vi "Main.vi"() -> ()   [LabVIEW 2015]
doc: "This template is for the Queued Message Handler design pattern.\n\nThe Event Handling Loop generates messages based on user interface actions.\n\nThe Message Handling Loop processes messages generated by the Event Handling Loop, or by other messages. The messages are string values, so new messages can be added easily to the Message Cases case structure in the Message Handling Loop. Each message cluster can also provide an optional value for Message Data, which is a variant that can be converted to whatever message-specific data is required."
uses:
  controls/UI Data.ctl
  support/Message Queue/Message Queue.lvlib
  support/User Event - Stop/User Event - Stop.lvlib
panel:
  out "Display <Replace Me>":string
  in  "Do Something Else <Replace Me>":bool
  in  "Do Something <Replace Me>":bool
  in  "Stop Button":bool
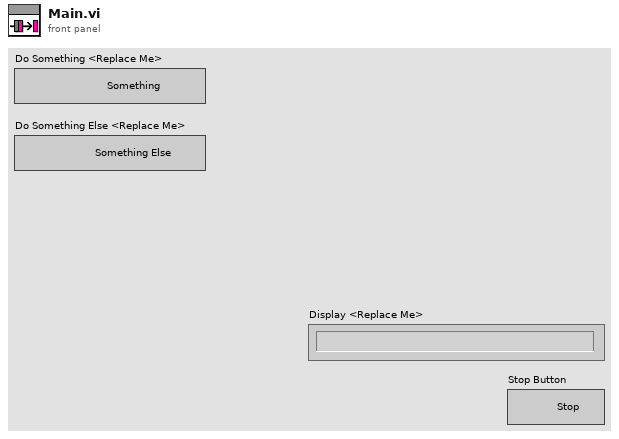
[diagram p1: front panel]
types:
  T1 = typedef "UI Data.ctl" = cluster{"Boolean <Replace Me>":bool, "String <Replace Me>":string, "Numeric <Replace Me>":dbl, "Do Something Ref":refnum<vi>, "Do Something Else Ref":refnum<vi>, "Data Display Ref":refnum<vi>, "Stop Button Ref":refnum<vi>}
  T2 = typedef "Message Queue.lvlib/All Message Queues.ctl" = cluster{"MHL":refnum<queue>, "Boiler controller":refnum<queue>}
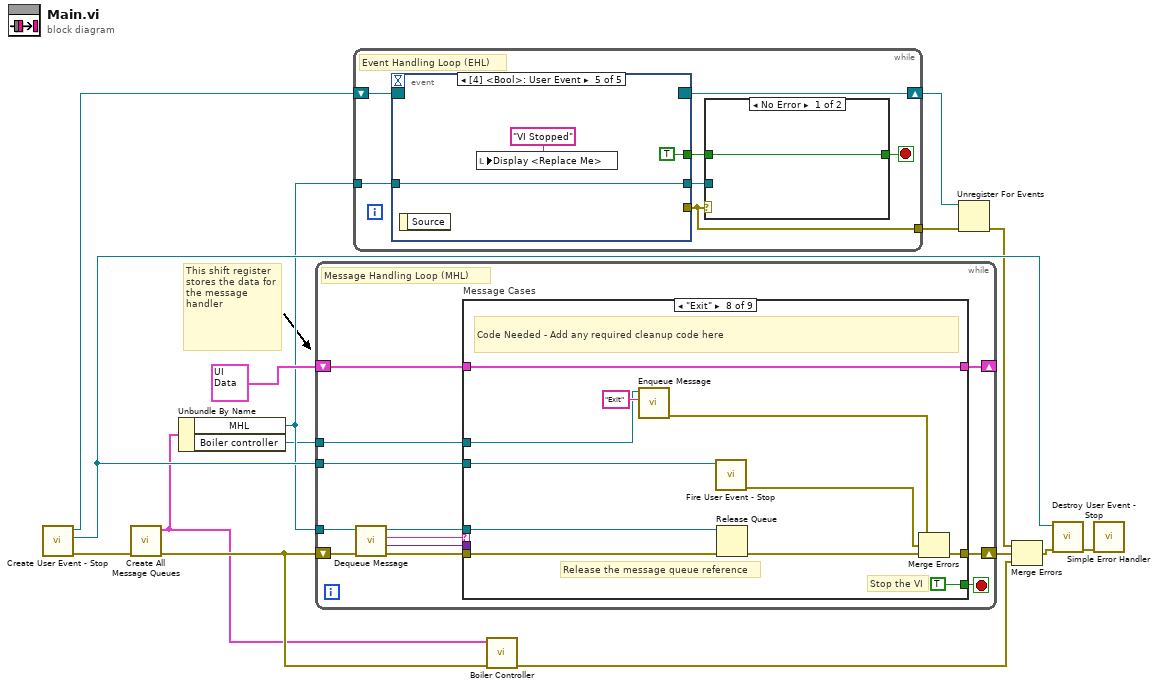
[diagram p0: block diagram]
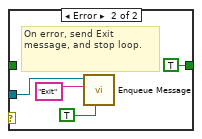
[diagram p2: hidden frame]
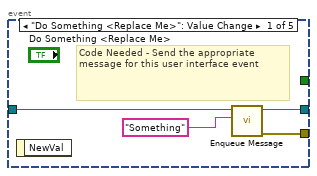
[diagram p3: hidden frame]
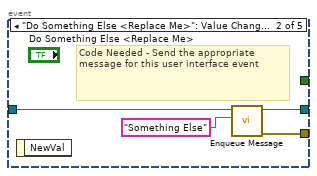
[diagram p4: hidden frame]
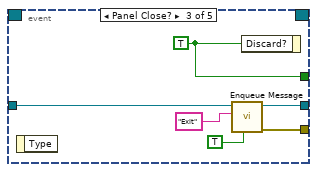
[diagram p5: hidden frame]
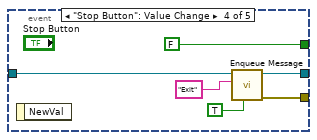
[diagram p6: hidden frame]
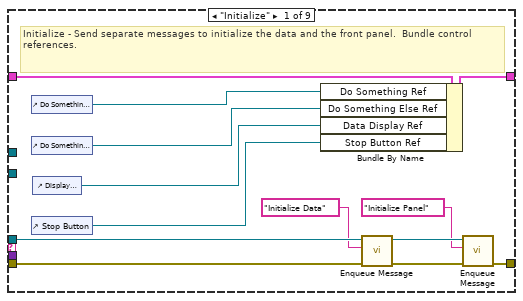
[diagram p7: hidden frame]
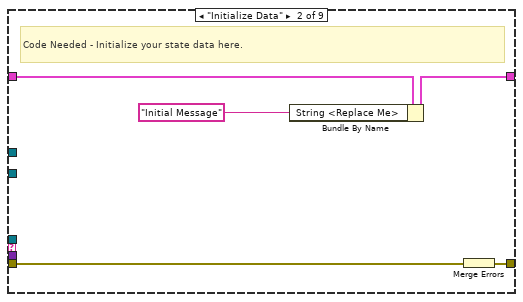
[diagram p8: hidden frame]
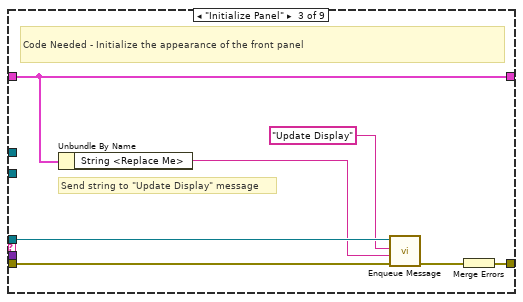
[diagram p9: hidden frame]
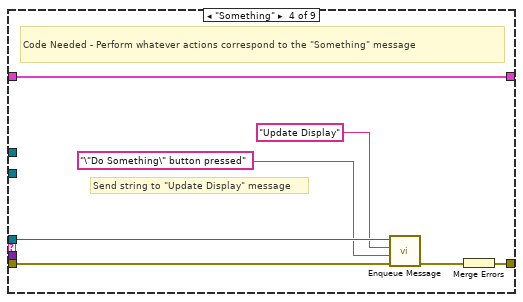
[diagram p10: hidden frame]
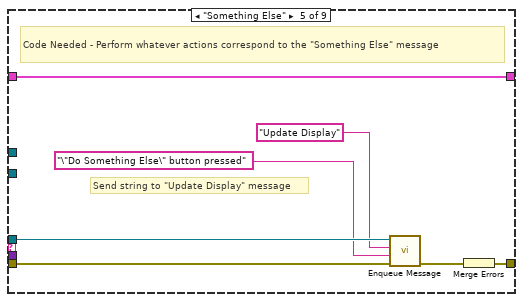
[diagram p11: hidden frame]
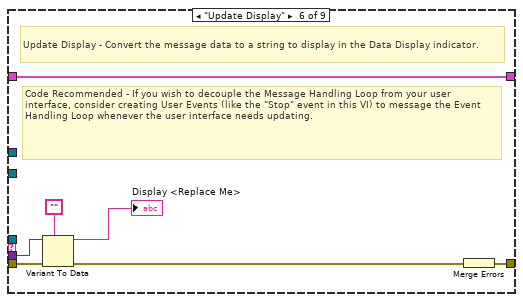
[diagram p12: hidden frame]
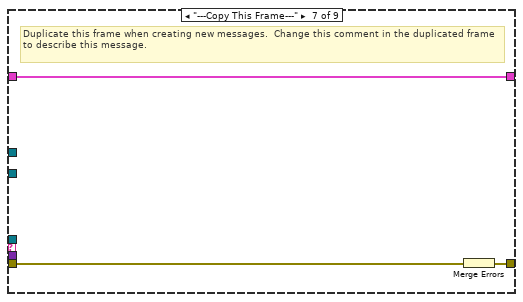
[diagram p13: hidden frame]
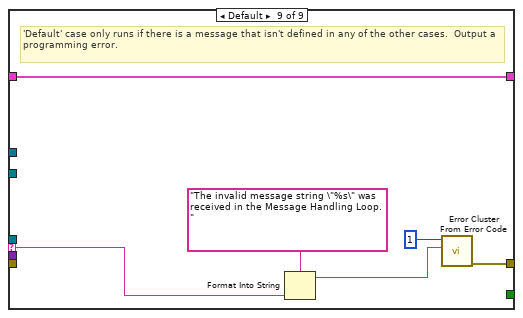
[diagram p14: hidden frame]
diagram:
  # "This shift register\nstores the data for the message handler"
  n1 = call "Create User Event - Stop.vi"() -> ("error out"=w14:errorcluster, "User bool - Stop"=w11:refnum<user-event>, "Event Registration Refnum"=w6:refnum<event-registration>)  [unwired: 9 in]
  n2 = call "Create All Message Queues.vi"("error in (no error)"=w14) -> ("error out"=w5:errorcluster, "Message Queues out"=w2:T2)  [unwired: 9 in]
  n3 = Unbundle By Name(w2) -> ("MHL"=w4:refnum<queue>, "Boiler controller"=w3:refnum<queue>)
  n4 = while {
    tunnel: w4 -> [w17]
    shift-right: [w26] -> _
    shift-left: T1 {"Boolean <Replace Me>"=TRUE, "String <Replace Me>"="", "Numeric <Replace Me>"=0.0, "Do Something Ref"=refnum, "Do Something Else Ref"=refnum, "Data Display Ref"=refnum, "Stop Button Ref"=refnum} ("Data Cluster") -> [w27]
    tunnel: w11 -> [w23]
    shift-right: [w24] -> w15
    shift-left: w5 -> [w22]
    tunnel: w3 -> [w16]
    stop <- w25 stop-if-true
    # "Message Handling Loop (MHL)"
    n5 = call "Dequeue Message.vi"("error in (no error)"=w22, "Message Queue"=w17) -> ("error out"=w21:errorcluster, "Message Data"=w19:variant, "Message"=w20:string, "dup Message Queue"=w18:refnum<queue>)  [unwired: 6 in]
    n6 = case "Message Cases" shown="\"Exit\"" w20 {
      selector: w20 -> [_ _ _ _ _ _ _ _ w91]
      tunnel: w18 -> [w36 _ w49 w55 w62 _ _ w87 _]
      tunnel: w21 -> [w39 w45 w50 w57 w64 w71 w76 w82 _]
      tunnel: [w40 w41 w51 w58 w65 w72 w74 w83 w89] -> w24
      tunnel: w27 -> [w33 w44 w52 w59 w66 w73 w75 w86 w93]
      tunnel: [w32 w43 w52 w59 w66 w73 w75 w86 w93] -> w26
      tunnel: [_ _ _ _ _ _ _ TRUE _] -> w25
      tunnel: w19 -> [_ _ _ _ _ w70 _ _ _]
      tunnel: w23 -> [_ _ _ _ _ _ _ w81 _]
      tunnel: w16 -> [_ _ _ _ _ _ _ w78 _]
      frame "Initialize" {
        # "Initialize - Send separate messages to initialize the data and the front panel.  Bundle control references."
        n7 = control-ref of="Do Something <Replace Me>"() -> (w31:refnum<vi>)
        n8 = control-ref of="Do Something Else <Replace Me>"() -> (w30:refnum<vi>)
        n9 = control-ref of="Stop Button"() -> (w28:refnum<vi>)
        n10 = control-ref of="Display <Replace Me>"() -> (w29:refnum<vi>)
        n11 = Bundle By Name(cluster=w33, "Do Something Ref"=w31, "Do Something Else Ref"=w30, "Data Display Ref"=w29, "Stop Button Ref"=w28) -> (w32:T1)
        n12 = call "Enqueue Message.vi"("error in (no error)"=w39, "Message"="Initialize Data", "Message Queue"=w36) -> ("error out"=w38:errorcluster, "dup Message Queue"=w37:refnum<queue>)  [unwired: 7 in]
        n13 = call "Enqueue Message.vi"("error in (no error)"=w38, "Message"="Initialize Panel", "Message Queue"=w37) -> ("error out"=w40:errorcluster)  [unwired: 7 in, 1 out]
      }
      frame "Initialize Data" {
        # "Code Needed - Initialize your state data here."
        n14 = Bundle By Name(cluster=w44, "String <Replace Me>"="Initial Message" ("Initial Message")) -> (w43:T1)
        n15 = Merge Errors(w45) -> (w41:errorcluster)
      }
      frame "Initialize Panel" {
        # "Send string to \"Update Display\" message"
        # "Code Needed - Initialize the appearance of the front panel"
        n16 = Unbundle By Name(w52) -> ("String <Replace Me>"=w46:string)
        n17 = call "Enqueue Message.vi"("error in (no error)"=w50, "Message Data"=w46, "Message"="Update Display", "Message Queue"=w49) -> ("error out"=w48:errorcluster)  [unwired: 6 in, 1 out]
        n18 = Merge Errors(w48) -> (w51:errorcluster)
      }
      frame "Something" {
        # "Send string to \"Update Display\" message"
        # "Code Needed - Perform whatever actions correspond to the \"Something\" message"
        n19 = call "Enqueue Message.vi"("error in (no error)"=w57, "Message Data"="\"Do Something\" button pressed" ("\"Do Something\" button pressed"), "Message"="Update Display", "Message Queue"=w55) -> ("error out"=w56:errorcluster)  [unwired: 6 in, 1 out]
        n20 = Merge Errors(w56) -> (w58:errorcluster)
      }
      frame "Something Else" {
        # "Send string to \"Update Display\" message"
        # "Code Needed - Perform whatever actions correspond to the \"Something Else\" message"
        n21 = call "Enqueue Message.vi"("error in (no error)"=w64, "Message Data"="\"Do Something Else\" button pressed" ("\"Do Something Else\" button pressed"), "Message"="Update Display", "Message Queue"=w62) -> ("error out"=w63:errorcluster)  [unwired: 6 in, 1 out]
        n22 = Merge Errors(w63) -> (w65:errorcluster)
      }
      frame "Update Display" {
        # "Code Recommended - If you wish to decouple the Message Handling Loop from your user interface, consider creating User Events (like the \"Stop\" event in this VI) to message the Event Handling Loop whenever the user interface needs updating."
        # "Update Display - Convert the message data to a string to display in the Data Display indicator."
        n23 = Variant To Data(error in=w71, type="", Variant=w70) -> (data=→"Display <Replace Me>":string, error out=w68:errorcluster)
        n24 = Merge Errors(w68) -> (w72:errorcluster)
      }
      frame "---Copy This Frame---" {
        # "Duplicate this frame when creating new messages.  Change this comment in the duplicated frame to describe this message."
        n25 = Merge Errors(w76) -> (w74:errorcluster)
      }
      frame "Exit" {
        # "Stop the VI"
        # "Release the message queue reference"
        # "Code Needed - Add any required cleanup code here"
        n26 = call "Enqueue Message.vi"("Message"="Exit", "Message Queue"=w78) -> ("error out"=w77:errorcluster)  [unwired: 8 in, 1 out]
        n27 = call "Fire User Event - Stop.vi"("User Event - Stop"=w81) -> ("error out"=w80:errorcluster)  [unwired: 10 in]
        n28 = Release Queue(queue=w87, error in (no error)=w82) -> (error out=w84:errorcluster)  [unwired: 1 in, 2 out]
        n29 = Merge Errors(w77, w80, w84) -> (w83:errorcluster)
      }
      frame Default {
        # "'Default' case only runs if there is a message that isn't defined in any of the other cases.  Output a programming error."
        n30 = Format Into String(format string="The invalid message string \"%s\" was received in the Message Handling Loop." ("Unknown Message Error Text"), w91) -> (resulting string=w88:string)  [unwired: 2 in, 1 out]
        n31 = call <vilib>:"Error Cluster From Error Code.vi"("error message (\"\")"=w88, "error code (0)"=1) -> ("error out"=w89:errorcluster)  [unwired: 7 in]
      }
    }
  }
  n32 = while {
    tunnel: w4 -> [w100]
    tunnel: [w96] -> w9
    shift-right: [w95] -> w8
    shift-left: w6 -> [w94]
    stop <- w98 stop-if-true
    # "Event Handling Loop (EHL)"
    n33 = event shown="[4] <Bool>: User Event" {
      selector: w94 -> [_ _ _ _ _]
      dyn-events: [_ _ _ _ _] -> w95
      timeout: _ -> [_ _ _ _ _]
      tunnel: [_ _ w119 FALSE ("Discard?") TRUE ("Discard?")] -> w99
      tunnel: w100 -> [w109 w113 w118 w125 w128]
      tunnel: [w108 w111 w117 w124 _] -> w96
      tunnel: [w107 w112 w116 w122 w128] -> w97
      event "Do Something <Replace Me>": Value Change {
        # "Code Needed - Send the appropriate message for this user interface event"
        n34 = event-data() -> ()  [unwired: 1 in, 1 out]
        n35 = call "Enqueue Message.vi"("Message"="Something", "Message Queue"=w109) -> ("error out"=w108:errorcluster, "dup Message Queue"=w107:refnum<queue>)  [unwired: 8 in]
      }
      event "Do Something Else <Replace Me>": Value Change {
        # "Code Needed - Send the appropriate message for this user interface event"
        n36 = event-data() -> ()  [unwired: 1 in, 1 out]
        n37 = call "Enqueue Message.vi"("Message"="Something Else", "Message Queue"=w113) -> ("error out"=w111:errorcluster, "dup Message Queue"=w112:refnum<queue>)  [unwired: 8 in]
      }
      event Panel Close? {
        w119 = TRUE ("Discard?")
        n38 = event-data() -> ()  [unwired: 1 in, 1 out]
        n39 = call "Enqueue Message.vi"("Priority Message? (F)"=TRUE, "Message"="Exit", "Message Queue"=w118) -> ("error out"=w117:errorcluster, "dup Message Queue"=w116:refnum<queue>)  [unwired: 7 in]
        n40 = event-data("Discard?"=w119) -> ()  [unwired: 1 in, 1 out]
      }
      event "Stop Button": Value Change {
        n41 = event-data() -> ()  [unwired: 1 in, 1 out]
        n42 = call "Enqueue Message.vi"("Priority Message? (F)"=TRUE, "Message"="Exit", "Message Queue"=w125) -> ("error out"=w124:errorcluster, "dup Message Queue"=w122:refnum<queue>)  [unwired: 7 in]
      }
      event User Event {
        n43 = event-data() -> ()  [unwired: 1 in, 1 out]
        n44 = local write "Display <Replace Me>"("VI Stopped" ("VI Stopped")) -> ()
      }
    }
    n45 = case shown="No Error" w96 {
      tunnel: [w101 TRUE ("Discard?")] -> w98
      tunnel: w99 -> [w101 _]
      tunnel: w97 -> [_ w104]
      frame No Error {
      }
      frame Error {
        # "On error, send Exit message, and stop loop."
        n46 = call "Enqueue Message.vi"("Priority Message? (F)"=TRUE, "Message"="Exit", "Message Queue"=w104) -> ()  [unwired: 7 in, 2 out]
      }
    }
  }
  n47 = call "Boiler Controller.vi"("error in (no error)"=w5, "Message Queues"=w2) -> ("error out"=w1:errorcluster)  [unwired: 9 in]
  n48 = Unregister For Events(event registration refnum=w8, error in=w9) -> (error out=w10:errorcluster)
  n49 = Merge Errors(w10, w15, w1) -> (w12:errorcluster)
  n50 = call "Destroy User Event - Stop.vi"("error in (no error)"=w12, "User Event - Stop"=w11) -> ("error out"=w13:errorcluster)  [unwired: 9 in]
  n51 = call <vilib>:"Simple Error Handler.vi"("error in (no error)"=w13) -> ()  [unwired: 4 in, 5 out]
